vi "Example.vi"() -> ()   [LabVIEW 2014, in "Meerstetter Lib.lvlib" / "Meerstetter TEC.lvclass"]
uses:
  Meerstetter TEC.lvclass
  reusable/Session APIs/File Access/Config Data/Config Session.ctl
  reusable/Session APIs/File Access/Config Data/Config Data.lvclass
  reusable/Session APIs/Session Log/System Log.lvclass
  reusable/Session APIs/Session Log/System Log.lvclass/System Log.ctl
  reusable/Session APIs/File Access/Config Data/Config Data.lvclass/Config Data.ctl
  Configurable Device/Configurable Device.lvclass/Configurable Device.ctl
  Data/mTEC Data.lvclass
  Data/mTEC Data.lvclass/mTEC Data.ctl
  Configurable Device/Write Handle.vi
  Configurable Device/Write Log Session.vi
  Configurable Device/Write ID.vi
  Data/Read Tobj.vi
  Data/Read Vout.vi
  reusable/Session APIs/Session Log/Accessors/Write Main Path.vi
  reusable/Session APIs/File Access/Config Data/Accessors/Write Cfg Path.vi
  <userlib>/_Session Fwk/Session - Root.lvclass
panel:
  out "Voltage":dbl(graph)
  out "Temperature":dbl(graph)
  in  "V (V)":dbl
  in  "I (A)":dbl
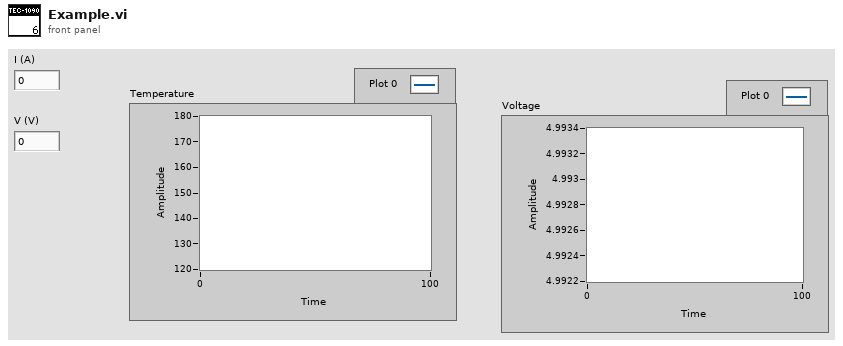
[diagram p1: front panel]
types:
  T1 = typedef "Config Data.lvclass/Config Session.ctl" = refnum<data-value>
  T2 = typedef "Session - Root.lvclass/Session Handle.ctl" = refnum<data-value>
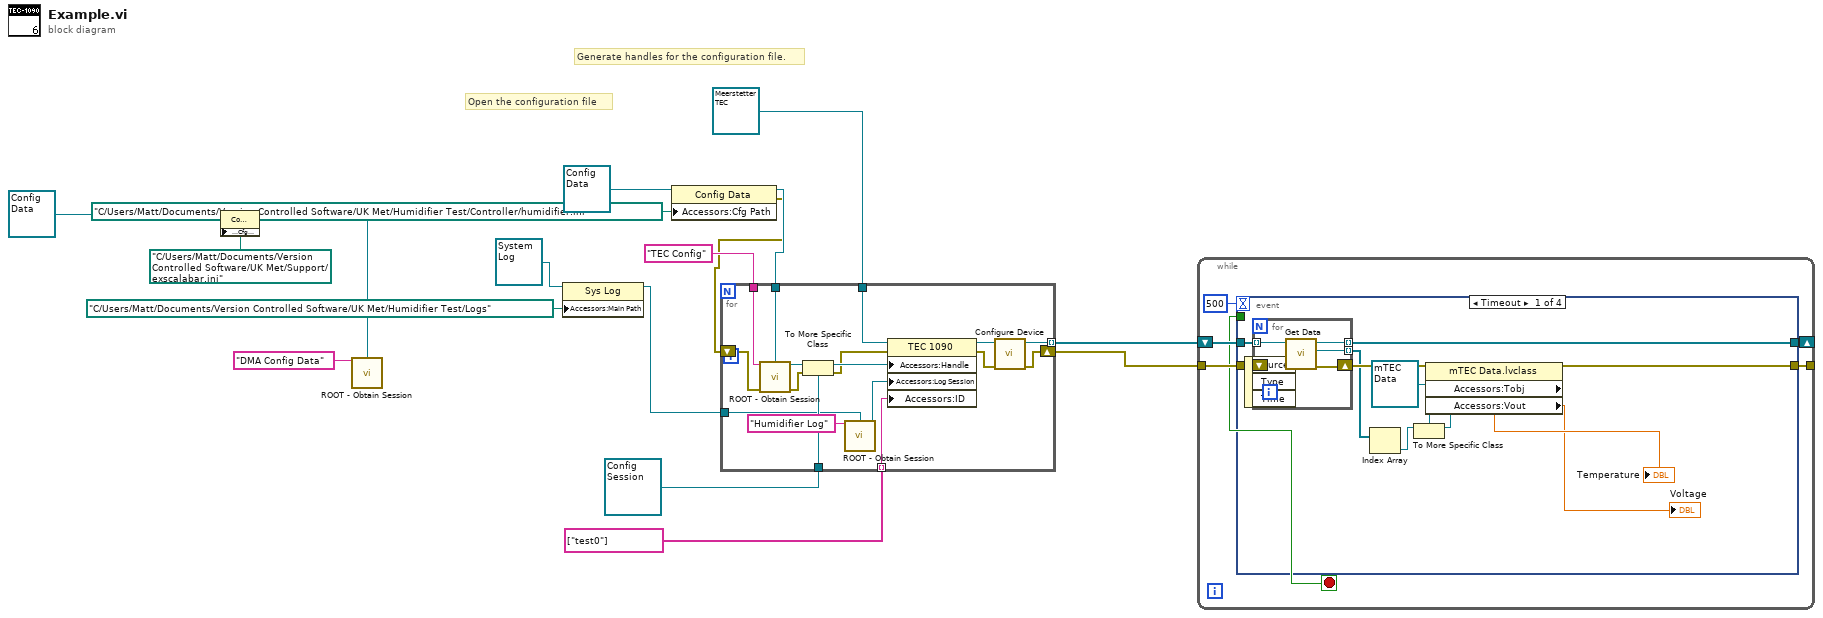
[diagram p0: block diagram]
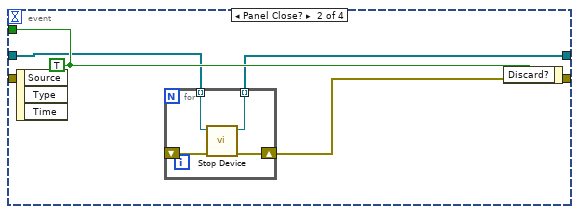
[diagram p2: hidden frame]
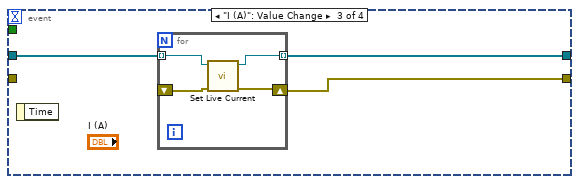
[diagram p3: hidden frame]
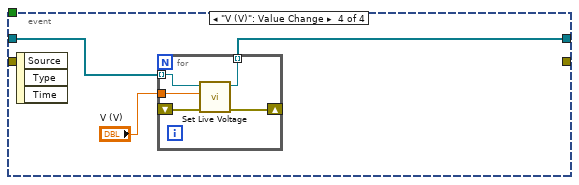
[diagram p4: hidden frame]
diagram:
  # "Open the configuration file"
  # "Generate handles for the configuration file."
  n1 = property class="Config Data"(reference=refnum<class "Config Data.lvclass"> refnum ("Config Data"), "Accessors:Cfg Path"=path "C:/Users/Matt/Documents/Version Controlled Software/UK Met/Support/exscalabar.ini" ("Path")) -> (reference out=w15:refnum<class "Config Data.lvclass">)  [unwired: 1 in, 1 out]
  n2 = call <userlib>:"ROOT - Obtain Session.vi"("Session Name ()"="DMA Config Data", "OBJ - Session"=w15) -> ()  [unwired: 11 in, 3 out]
  n3 = property class="Sys Log"(reference=refnum<class "System Log.lvclass"> refnum ("Sys Log"), "Accessors:Main Path"=path "C:/Users/Matt/Documents/Version Controlled Software/UK Met/Humidifier Test/Logs" ("Main Path")) -> (reference out=w1:refnum<class "System Log.lvclass">)  [unwired: 1 in, 1 out]
  n4 = property class="Config Data"(reference=refnum<class "Config Data.lvclass"> refnum ("Config Data"), "Accessors:Cfg Path"=path "C:/Users/Matt/Documents/Version Controlled Software/UK Met/Humidifier Test/Controller/humidifier.ini" ("Cfg Path")) -> (reference out=w5:refnum<class "Config Data.lvclass">, error out=w4:errorcluster)  [unwired: 1 in]
  n5 = for {
    tunnel: [w32] -> w11 mode=indexing
    tunnel: refnum<class "Meerstetter TEC.lvclass"> refnum ("TEC 1090") -> [w34]
    shift-right: [w31] -> w10
    shift-left: w4 -> [w28]
    tunnel: string[] ["test0"] -> [w18] mode=indexing
    tunnel: T1 refnum ("Session Handle") -> [w27]
    tunnel: "TEC Config" ("Session Name ()") -> [w23]
    tunnel: w5 -> [w22]
    tunnel: w1 -> [w20]
    n6 = call <userlib>:"ROOT - Obtain Session.vi"("Session Name ()"=w23, "OBJ - Session"=w22, "error in (no error)"=w28) -> ("Session Handle"=w29:T2, "error out"=w25:errorcluster)  [unwired: 10 in, 1 out]
    n7 = To More Specific Class(target class=w27, reference=w29, error in=w25) -> (specific class reference=w26:T1, error out=w24:errorcluster)
    n8 = call <userlib>:"ROOT - Obtain Session.vi"("Session Name ()"="Humidifier Log", "OBJ - Session"=w20) -> ("Session Handle"=w21:T2)  [unwired: 11 in, 2 out]
    n9 = property class="TEC 1090"(reference=w34, error in=w24, "Accessors:Handle"=w26, "Accessors:Log Session"=w21, "Accessors:ID"=w18) -> (reference out=w33:refnum<class "Meerstetter TEC.lvclass">, error out=w30:errorcluster)
    n10 = call-dynamic "Configure Device.vi"("error in"=w30, "Meerstetter TEC in"=w33) -> ("error out"=w31:errorcluster, "Meerstetter TEC out"=w32:refnum<class "Meerstetter TEC.lvclass">)  [unwired: 7 in, 1 out]
  }
  n11 = while {
    tunnel: w10 -> [w39]
    tunnel: [w38] -> _
    shift-right: [w36] -> _
    shift-left: w11 -> [w40]
    stop <- w37 stop-if-true
    n12 = event shown="[0] Timeout" {
      selector: _ -> [_ _ _ _]
      dyn-events: _ -> [_ _ _ _]
      timeout: 500 -> [_ _ _ _]
      tunnel: w40 -> [w50 w58 w66 w73]
      tunnel: w39 -> [w49 _ _ _]
      tunnel: [w48 w56 w64 _] -> w38
      tunnel: [_ w59 _ _] -> w37
      tunnel: [w47 w57 w65 w72] -> w36
      event Timeout {
        n13 = event-data() -> ()  [unwired: 1 in, 3 out]
        n14 = for {
          tunnel: w50 -> [w55] mode=indexing
          shift-right: [w53] -> w48
          shift-left: w49 -> [w54]
          tunnel: [w52] -> w46 mode=indexing
          tunnel: [w51] -> w47 mode=indexing
          n15 = call-dynamic "Get Data.vi"("error in"=w54, "Meerstetter TEC in"=w55) -> ("error out"=w53:errorcluster, "DataOut"=w52:refnum<class "Data.lvclass">, "Meerstetter TEC out"=w51:refnum<class "Meerstetter TEC.lvclass">)  [unwired: 7 in]
        }
        n16 = Index Array(array=w46) -> (element=w45:refnum<class "Data.lvclass">)  [unwired: 1 in]
        n17 = To More Specific Class(target class=refnum<class "mTEC Data.lvclass"> refnum ("Meerstetter Lib.lvlib:mTEC Data.lvclass"), reference=w45) -> (specific class reference=w43:refnum<class "mTEC Data.lvclass">)  [unwired: 1 in, 1 out]
        n18 = property class="mTEC Data.lvclass"(reference=w43) -> ("Accessors:Tobj"=→"Temperature":dbl, "Accessors:Vout"=→"Voltage":dbl)  [unwired: 1 in, 2 out]
      }
      event Panel Close? {
        w59 = TRUE ("Discard?")
        n19 = event-data() -> ()  [unwired: 1 in, 3 out]
        n20 = for {
          tunnel: w58 -> [w63] mode=indexing
          tunnel: [w62] -> w57 mode=indexing
          shift-right: [w61] -> w56
          shift-left: _ -> [w60]
          n21 = call-dynamic "Stop Device.vi"("error in"=w60, "Meerstetter TEC in"=w63) -> ("error out"=w61:errorcluster, "Meerstetter TEC out"=w62:refnum<class "Meerstetter TEC.lvclass">)  [unwired: 8 in]
        }
        n22 = event-data("Discard?"=w59) -> ()  [unwired: 1 in, 1 out]
      }
      event "I (A)": Value Change {
        n23 = event-data() -> ()  [unwired: 1 in, 1 out]
        n24 = for {
          tunnel: w66 -> [w70] mode=indexing
          tunnel: [w69] -> w65 mode=indexing
          shift-right: [w68] -> w64
          shift-left: _ -> [w67]
          n25 = call "Set Live Current.vi"("error in"=w67, "TEC 1090 in"=w70) -> ("error out"=w68:errorcluster, "TEC 1090 out"=w69:refnum<class "Meerstetter TEC.lvclass">)  [unwired: 8 in]
        }
      }
      event "V (V)": Value Change {
        n26 = event-data() -> ()  [unwired: 1 in, 3 out]
        n27 = for {
          tunnel: w73 -> [w78] mode=indexing
          tunnel: [w77] -> w72 mode=indexing
          shift-right: [w76] -> _
          shift-left: _ -> [w75]
          tunnel: "V (V)" -> [w74]
          n28 = call "Set Live Voltage.vi"("error in"=w75, "V"=w74, "TEC 1090 in"=w78) -> ("error out"=w76:errorcluster, "TEC 1090 out"=w77:refnum<class "Meerstetter TEC.lvclass">)  [unwired: 7 in]
        }
      }
    }
  }
